vi "PH_SHS_Analysis_Calibrator.get Cam instances.vi"(0 "i ref in":refnum<vi>, 5 "error in":errorcluster) -> (14 "i ref out":refnum<vi>, 19 "error out":errorcluster)   [LabVIEW 2014, in "PH_SHS_Analysis_Calibrator.lvlib"]
doc: "This VI gets the camaras instanciated locally and writes them to own attributes and the GUI element."
uses:
  PH_SHS_Analysis_Calibrator.lvlib
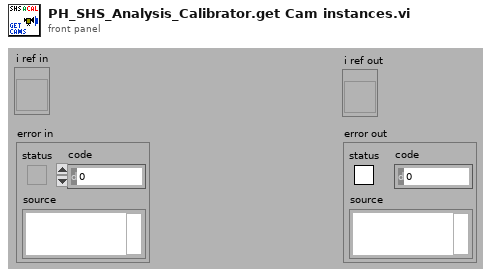
[diagram p1: front panel]
types:
  T1 = typedef "PH_SHS_Analysis_Calibrator.lvlib/PH_SHS_Analysis_Calibrator.i attribute.ctl" = cluster{"GUI Refs":cluster{"Available Cams":refnum<vi>, "OK":refnum<vi>, "Skip":refnum<vi>, "Repeat":refnum<vi>, "Cancel":refnum<vi>, "Dialog":refnum<vi>, "Enough Images?":refnum<vi>}, "Cam instances":string[], "Status":cluster{"#":i32, "Data calculated":bool, "Wanted #":i32}, "IMAQ Image Array":T2[], "Pixel Size [µm]":dbl, "MLA Pitch [µm]":dbl, "Method":enum16{"automatic", "manual"}, "Enough Images?":bool, "SHS Reference Result":T3, "Calculation Error":errorcluster}
  T2 = typedef "IMAQ Image.ctl" = refnum<image>
  T3 = typedef "SHS_Common.lvlib/SHSReference.ctl" = cluster{"Reference":T4[][], "Lens Array Pitch [px]":dbl}
  T4 = typedef "SHS_Common.lvlib/ReferencePoint.ctl" = cluster{"Rect":T5, "Point":T6}
  T5 = typedef "SHS_Common.lvlib/Rectangle.ctl" = cluster{"Left":i32, "Top":i32, "Right":i32, "Bottom":i32}
  T6 = typedef "SHS_Common.lvlib/Point.ctl" = cluster{"x":dbl, "y":dbl, "valid?":bool, "weight":dbl}
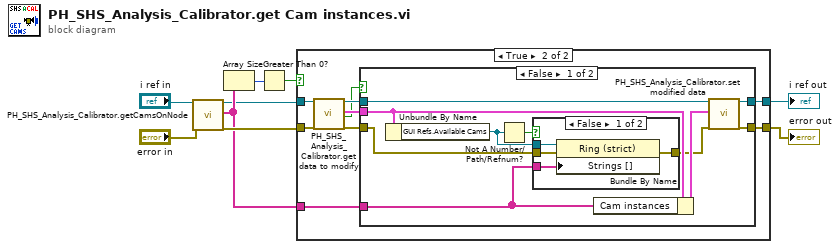
[diagram p0: block diagram]
diagram:
  n1 = call "PH_SHS_Analysis_Calibrator.getCamsOnNode.vi"("i ref in"="i ref in", "error in (no error)"="error in") -> ("i ref out"=w1:refnum<vi>, "cams on node"=w3:string[], "error out"=w7:errorcluster)  [unwired: 15 in]
  n2 = Array Size(array=w3) -> (size(s)=w6:i32)
  n3 = Greater Than 0?(x=w6) -> (x > 0?=w5:bool)
  n4 = case shown="True" w5 {
    tunnel: w7 -> [w11 w15]
    tunnel: [w11 w14] -> w9
    tunnel: w1 -> [w10 w13]
    tunnel: [w10 w16] -> w8
    tunnel: w3 -> [_ w12]
    frame False {
    }
    frame True {
      n5 = call "PH_SHS_Analysis_Calibrator.get data to modify.vi"("i ref in"=w13, "error in (no error)"=w15) -> ("i ref out"=w20:refnum<vi>, "i attribute"=w18:T1, "timed out"=w17:bool, "error out"=w19:errorcluster)  [unwired: 14 in]
      n6 = case shown="False" w17 {
        tunnel: w20 -> [w30 w37]
        tunnel: w19 -> [w24 w36]
        tunnel: [w29 w36] -> w14
        tunnel: [w28 w37] -> w16
        tunnel: w18 -> [w26 _]
        tunnel: w12 -> [w25 _]
        frame False {
          n7 = Unbundle By Name(w26) -> ("GUI Refs.Available Cams"=w21:refnum<vi>)
          n8 = Not A Number/Path/Refnum?(number/path/refnum=w21) -> (NaN/Path/Refnum?=w22:bool)
          n9 = case shown="False" w22 {
            tunnel: w21 -> [w34 _]
            tunnel: w25 -> [w33 _]
            tunnel: w24 -> [w32 w35]
            tunnel: [w31 w35] -> w23
            frame False {
              n10 = property class="Ring (strict)"(reference=w34, error in=w32, "Strings []"=w33) -> (error out=w31:errorcluster)  [unwired: 1 out]
            }
            frame True {
            }
          }
          n11 = Bundle By Name(cluster=w26, "Cam instances"=w25) -> (w27:T1)
          n12 = call "PH_SHS_Analysis_Calibrator.set modified data.vi"("i ref in"=w30, "i attribute"=w27, "error in (no error)"=w23) -> ("i ref out"=w28:refnum<vi>, "error out"=w29:errorcluster)  [unwired: 15 in]
        }
        frame True {
        }
      }
    }
  }
  "i ref out" <- w8
  "error out" <- w9
